vi "Replace Analysis Cluster.vi"() -> (0 "error out":errorcluster, 4 "Path":path)   [LabVIEW 2020]
panel:
  in  "OK Button":bool
  in  "stop":bool
  out "String":string
  in  "Correct Meas setup file":path
  in  "Analysis Cluster to Inject":string[][](array[string])=[["Inst Array", "Port", "Inst type", "Units symbol", "Sampling Rate (Hz)", "Device ID", "Sync Delay (ms)", "Ch No", "Use latest Calib", "Calib filename", "Label", "X Pos", "Y Pos", "Z Pos", "Initial X", "Initial Y", "Initial Z", "Traverse Setup", "On Axes", "ADAM_Ch_Name", "Code name", "Metadata Ch Names", "Metadata Ch Values"], ["LDA", "", "LDA Vel", "U", "250.00", "LDA_IP.vi", "0.00", "0", "FALSE", "", "", "80.000", "0.000", "-105.002", "0.000", "0.000", "0.000", "Aero_Enclosure", "X Y Z", "", "1LDA:U", "", ""], ["LDA", "", "LDA Vel", "W", "250.00", "LDA_IP.vi", "0.00", "1", "FALSE", "", "", "0.000", "0.000", "0.000", "0.000", "0.000", "0.000", "Position N/A", "X Y Z", "", "2LDA:U", "", ""], ["Analogue", "COM18", "Raw with zero offsetting", "N01", "800.00", "Pressure_Multiplexer.vi", "0.00", "0", "FALSE", "", "N01", "0.000", "0.000", "1.000", "0.000", "0.000", "1.000", "No Traverse", "X Y Z", "", "1RZ:U", "", ""], ["Analogue", "COM18", "Raw with zero offsetting", "N02", "800.00", "Pressure_Multiplexer.vi", "0.00", "1", "FALSE", "", "N02", "0.004", "0.013", "1.000", "0.004", "0.013", "1.000", "No Traverse", "X Y Z", "", "2RZ:U", "", ""], ["Analogue", "COM18", "Raw with zero offsetting", "N04", "800.00", "Pressure_Multiplexer.vi", "0.00", "2", "FALSE", "", "N04", "0.015", "0.025", "1.000", "0.015", "0.025", "1.000", "No Traverse", "X Y Z", "", "3RZ:U", "", ""], ["Analogue", "COM18", "Raw with zero offsetting", "N06", "800.00", "Pressure_Multiplexer.vi", "0.00", "3", "FALSE", "", "N06", "0.032", "0.037", "1.000", "0.032", "0.037", "1.000", "No Traverse", "X Y Z", "", "4RZ:U", "", ""], ["Analogue", "COM18", "Raw with zero offsetting", "N07", "800.00", "Pressure_Multiplexer.vi", "0.00", "4", "FALSE", "", "N07", "0.057", "0.047", "1.000", "0.057", "0.047", "1.000", "No Traverse", "X Y Z", "", "5RZ:U", "", ""], ["Analogue", "COM18", "Raw with zero offsetting", "N09", "800.00", "Pressure_Multiplexer.vi", "0.00", "5", "FALSE", "", "N09", "0.089", "0.056", "1.000", "0.089", "0.056", "1.000", "No Traverse", "X Y Z", "", "6RZ:U", "", ""], ["Analogue", "COM18", "Raw with zero offsetting", "N10", "800.00", "Pressure_Multiplexer.vi", "0.00", "6", "FALSE", "", "N10", "0.126", "0.063", "1.000", "0.126", "0.063", "1.000", "No Traverse", "X Y Z", "", "7RZ:U", "", ""], ["Analogue", "COM18", "Raw with zero offsetting", "N11", "800.00", "Pressure_Multiplexer.vi", "0.00", "7", "FALSE", "", "N11", "0.168", "0.069", "1.000", "0.168", "0.069", "1.000", "No Traverse", "X Y Z", "", "8RZ:U", "", ""], ["Analogue", "COM18", "Raw with zero offsetting", "N13", "800.00", "Pressure_Multiplexer.vi", "0.00", "8", "FALSE", "", "N13", "0.216", "0.073", "1.000", "0.216", "0.073", "1.000", "No Traverse", "X Y Z", "", "9RZ:U", "", ""], ["Analogue", "COM18", "Raw with zero offsetting", "N14", "800.00", "Pressure_Multiplexer.vi", "0.00", "34", "FALSE", "", "N14", "0.268", "0.075", "1.000", "0.268", "0.075", "1.000", "No Traverse", "X Y Z", "", "10RZ:U", "", ""], ["Analogue", "COM18", "Raw with zero offsetting", "N15", "800.00", "Pressure_Multiplexer.vi", "0.00", "10", "FALSE", "", "N15", "0.323", "0.075", "1.000", "0.323", "0.075", "1.000", "No Traverse", "X Y Z", "", "11RZ:U", "", ""], ["Analogue", "COM18", "Raw with zero offsetting", "N16", "800.00", "Pressure_Multiplexer.vi", "0.00", "11", "FALSE", "", "N16", "0.380", "0.073", "1.000", "0.380", "0.073", "1.000", "No Traverse", "X Y Z", "", "12RZ:U", "", ""], ["Analogue", "COM18", "Raw with zero offsetting", "N18", "800.00", "Pressure_Multiplexer.vi", "0.00", "12", "FALSE", "", "N18", "0.440", "0.070", "1.000", "0.440", "0.070", "1.000", "No Traverse", "X Y Z", "", "13RZ:U", "", ""], ["Analogue", "COM18", "Raw with zero offsetting", "N19", "800.00", "Pressure_Multiplexer.vi", "0.00", "13", "FALSE", "", "N19", "0.500", "0.066", "1.000", "0.500", "0.066", "1.000", "No Traverse", "X Y Z", "", "14RZ:U", "", ""], ["Analogue", "COM18", "Raw with zero offsetting", "N20", "800.00", "Pressure_Multiplexer.vi", "0.00", "14", "FALSE", "", "N20", "0.587", "0.058", "1.000", "0.587", "0.058", "1.000", "No Traverse", "X Y Z", "", "15RZ:U", "", ""], ["Analogue", "COM18", "Raw with zero offsetting", "N22", "800.00", "Pressure_Multiplexer.vi", "0.00", "15", "FALSE", "", "N22", "0.671", "0.049", "1.000", "0.671", "0.049", "1.000", "No Traverse", "X Y Z", "", "16RZ:U", "", ""], ["Analogue", "COM18", "Raw with zero offsetting", "N23", "800.00", "Pressure_Multiplexer.vi", "0.00", "16", "FALSE", "", "N23", "0.750", "0.040", "1.000", "0.750", "0.040", "1.000", "No Traverse", "X Y Z", "", "17RZ:U", "", ""], ["Analogue", "COM18", "Raw with zero offsetting", "N24", "800.00", "Pressure_Multiplexer.vi", "0.00", "17", "FALSE", "", "N24", "0.821", "0.030", "1.000", "0.821", "0.030", "1.000", "No Traverse", "X Y Z", "", "18RZ:U", "", ""], ["Analogue", "COM18", "Raw with zero offsetting", "N26", "800.00", "Pressure_Multiplexer.vi", "0.00", "18", "FALSE", "", "N26", "0.883", "0.021", "1.000", "0.883", "0.021", "1.000", "No Traverse", "X Y Z", "", "19RZ:U", "", ""], ["Analogue", "COM18", "Raw with zero offsetting", "N27", "800.00", "Pressure_Multiplexer.vi", "0.00", "19", "FALSE", "", "N27", "0.933", "0.013", "1.000", "0.933", "0.013", "1.000", "No Traverse", "X Y Z", "", "20RZ:U", "", ""], ["Analogue", "COM18", "Raw with zero offsetting", "N29", "800.00", "Pressure_Multiplexer.vi", "0.00", "20", "FALSE", "", "N29", "0.970", "0.007", "1.000", "0.970", "0.007", "1.000", "No Traverse", "X Y Z", "", "21RZ:U", "", ""], ["Analogue", "COM18", "Raw with zero offsetting", "N30", "800.00", "Pressure_Multiplexer.vi", "0.00", "21", "FALSE", "", "N30", "1.000", "0.000", "1.000", "1.000", "0.000", "1.000", "No Traverse", "X Y Z", "", "22RZ:U", "", ""], ["Analogue", "COM18", "Raw with zero offsetting", "N28", "800.00", "Pressure_Multiplexer.vi", "0.00", "22", "FALSE", "", "N28", "0.953", "-0.010", "-1.000", "0.953", "-0.010", "-1.000", "No Traverse", "X Y Z", "", "23RZ:U", "", ""], ["Analogue", "COM18", "Raw with zero offsetting", "N25", "800.00", "Pressure_Multiplexer.vi", "0.00", "23", "FALSE", "", "N25", "0.821", "-0.030", "-1.000", "0.821", "-0.030", "-1.000", "No Traverse", "X Y Z", "", "24RZ:U", "", ""], ["Analogue", "COM18", "Raw with zero offsetting", "N21", "800.00", "Pressure_Multiplexer.vi", "0.00", "24", "FALSE", "", "N21", "0.629", "-0.054", "-1.000", "0.629", "-0.054", "-1.000", "No Traverse", "X Y Z", "", "25RZ:U", "", ""], ["Analogue", "COM18", "Raw with zero offsetting", "N17", "800.00", "Pressure_Multiplexer.vi", "0.00", "25", "FALSE", "", "N17", "0.413", "-0.072", "-1.000", "0.413", "-0.072", "-1.000", "No Traverse", "X Y Z", "", "26RZ:U", "", ""], ["Analogue", "COM18", "Raw with zero offsetting", "N12", "800.00", "Pressure_Multiplexer.vi", "0.00", "26", "FALSE", "", "N12", "0.213", "-0.073", "-1.000", "0.213", "-0.073", "-1.000", "No Traverse", "X Y Z", "", "27RZ:U", "", ""], ["Analogue", "COM18", "Raw with zero offsetting", "N08", "800.00", "Pressure_Multiplexer.vi", "0.00", "27", "FALSE", "", "N08", "0.067", "-0.050", "-1.000", "0.067", "-0.050", "-1.000", "No Traverse", "X Y Z", "", "28RZ:U", "", ""], ["Analogue", "COM18", "Raw with zero offsetting", "N05", "800.00", "Pressure_Multiplexer.vi", "0.00", "28", "FALSE", "", "N05", "0.021", "-0.030", "-1.000", "0.021", "-0.030", "-1.000", "No Traverse", "X Y Z", "", "29RZ:U", "", ""], ["Analogue", "COM18", "Raw with zero offsetting", "N03", "800.00", "Pressure_Multiplexer.vi", "0.00", "29", "FALSE", "", "N03", "0.004", "-0.014", "-1.000", "0.004", "-0.014", "-1.000", "No Traverse", "X Y Z", "", "30RZ:U", "", ""], ["Analogue", "COM23", "Generic Polynomial", "D", "5000.00", "Na-DAS_7609.vi", "0.00", "0", "FALSE", "Z:\\2021\\Aero_Tunnel\\Haydn Wootton\\Calibrations\\Cal_12-2021\\Laser Disp Volts to Angle2.xls", "", "0.000", "0.000", "0.000", "0.000", "0.000", "0.000", "Position N/A", "X Y Z", "", "1Gen:U", "", ""], ["Analogue", "COM23", "Raw voltage", "Sync", "5000.00", "Na-DAS_7609.vi", "0.00", "1", "FALSE", "", "", "0.000", "0.000", "0.000", "0.000", "0.000", "0.000", "Position N/A", "X Y Z", "", "1RV:U", "", ""]]
  out "Array":path[](array[path])
  out "File Changed":bool
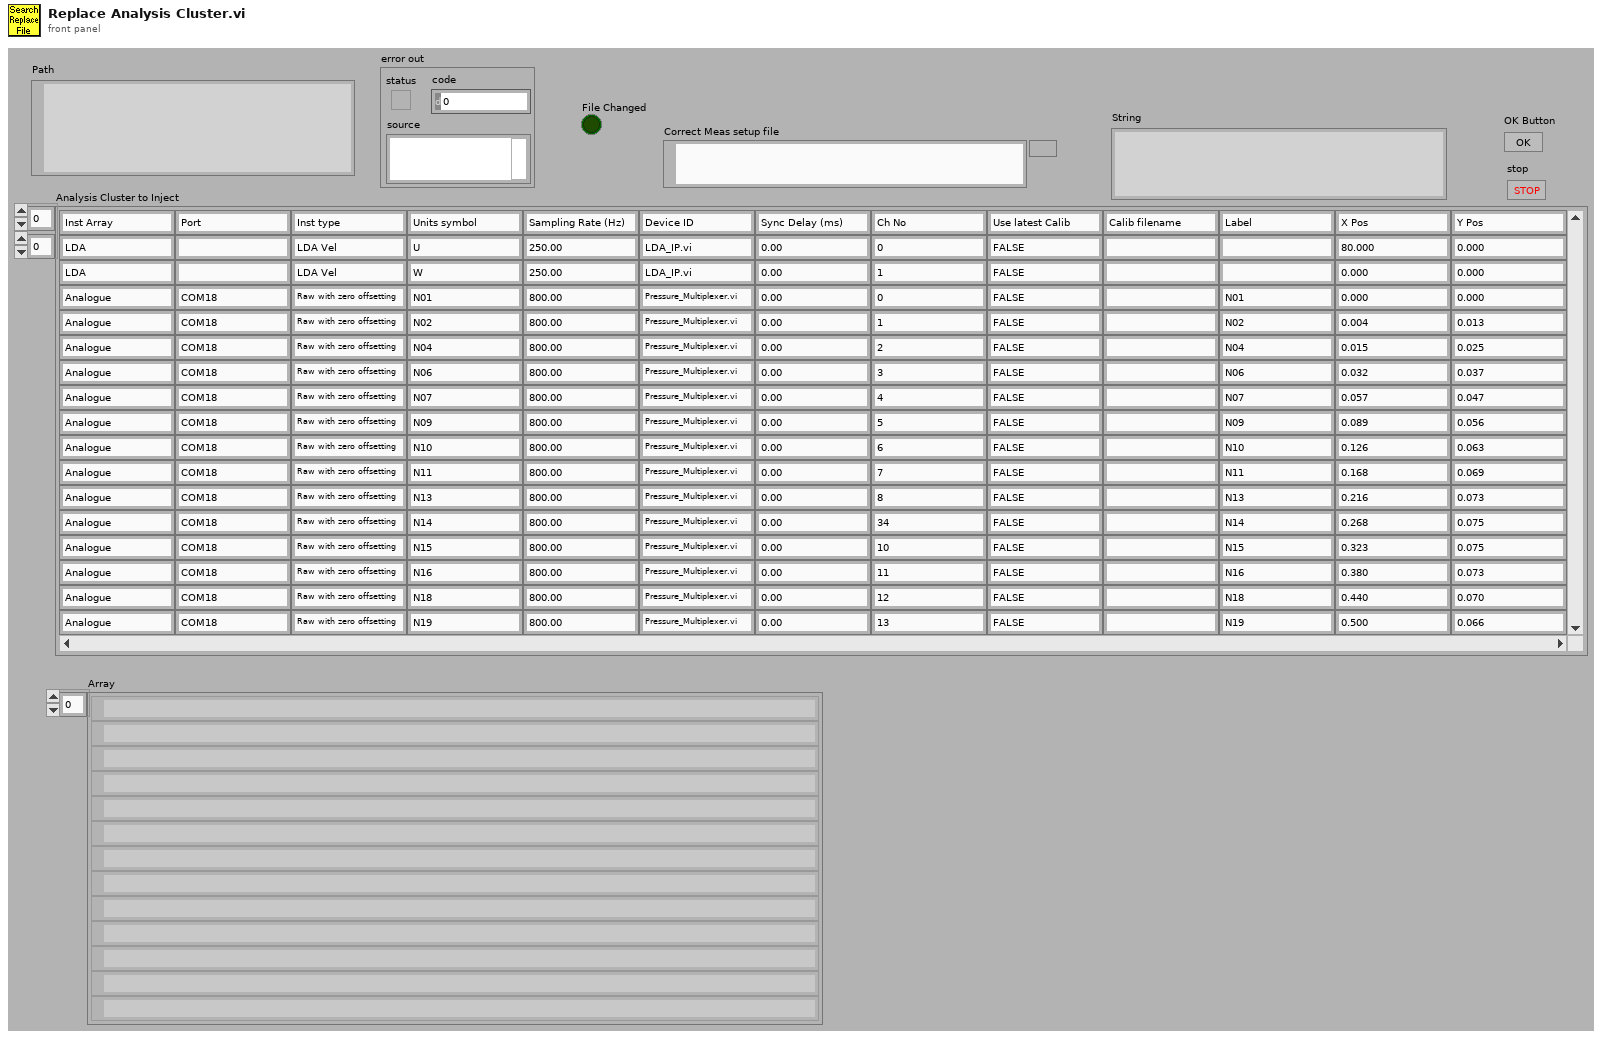
[diagram p1: front panel]
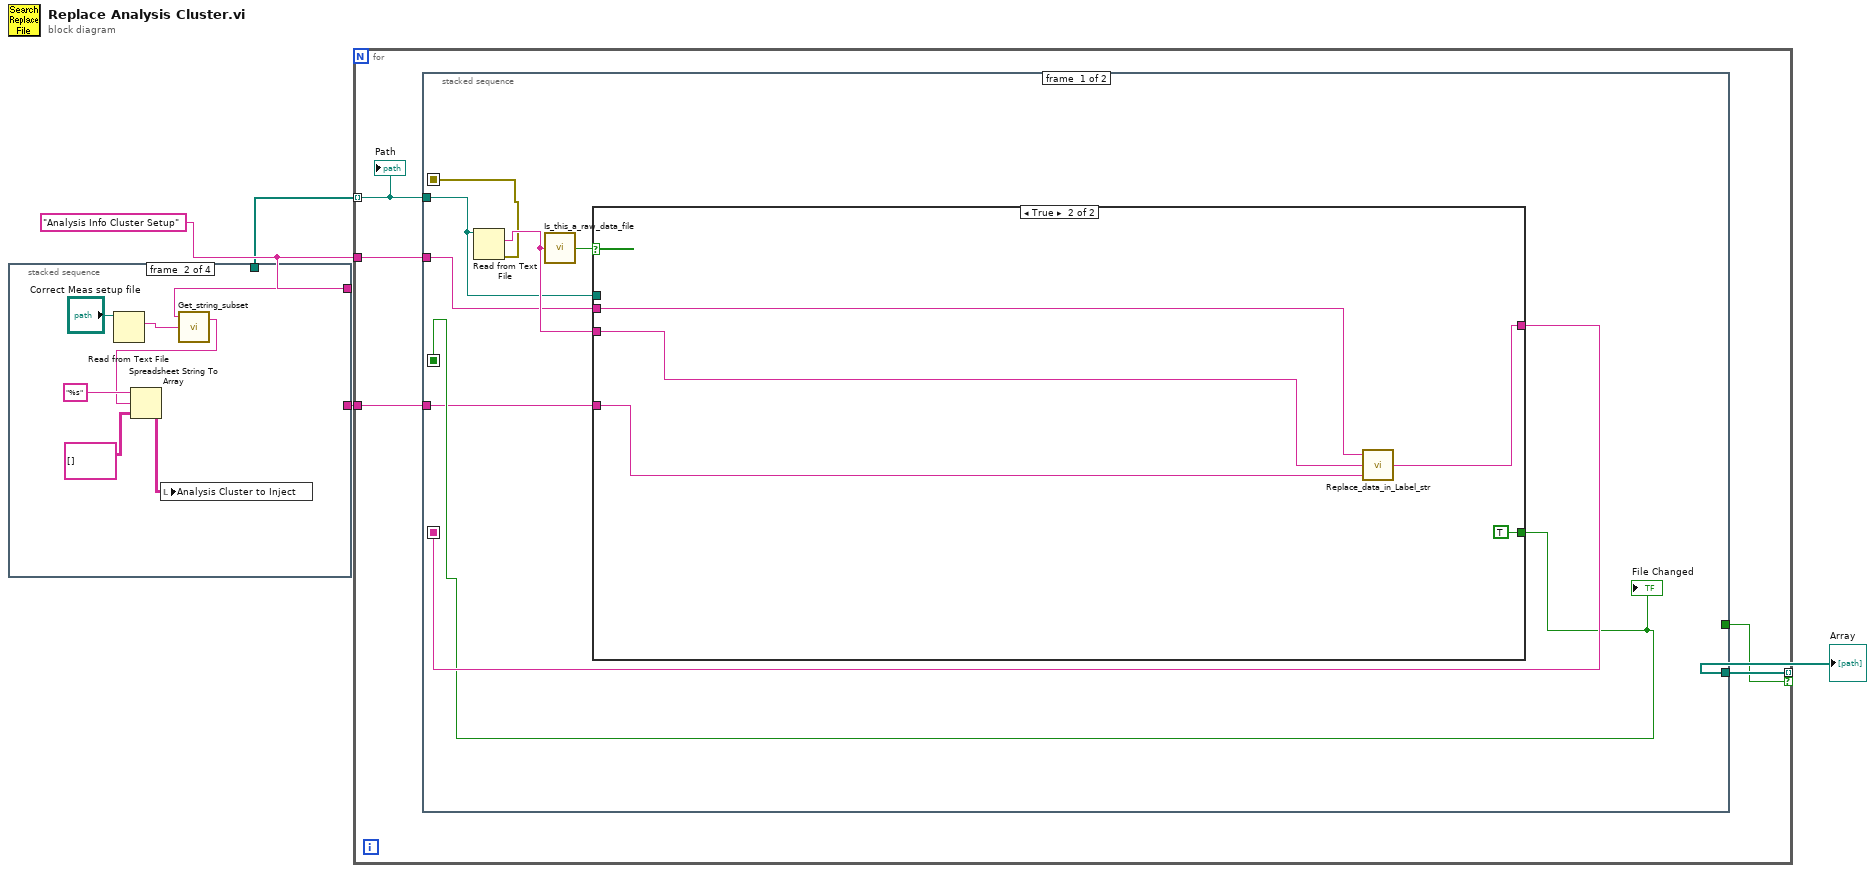
[diagram p0: block diagram]
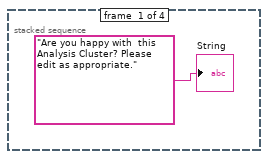
[diagram p2: hidden frame]
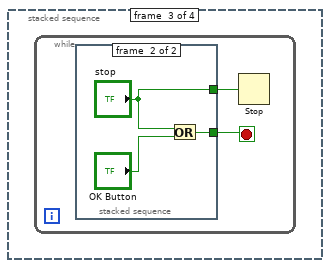
[diagram p3: hidden frame]
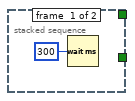
[diagram p4: hidden frame]
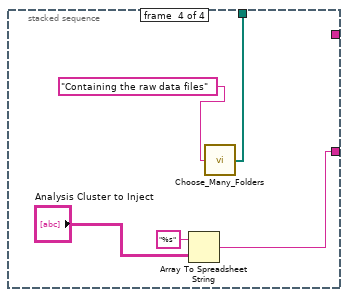
[diagram p5: hidden frame]
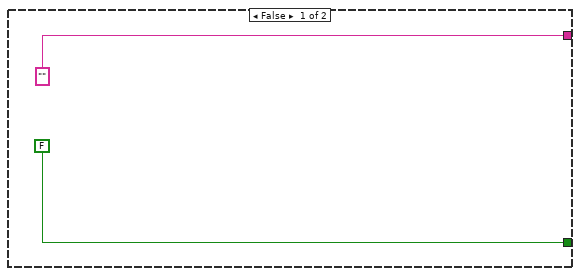
[diagram p6: hidden frame]
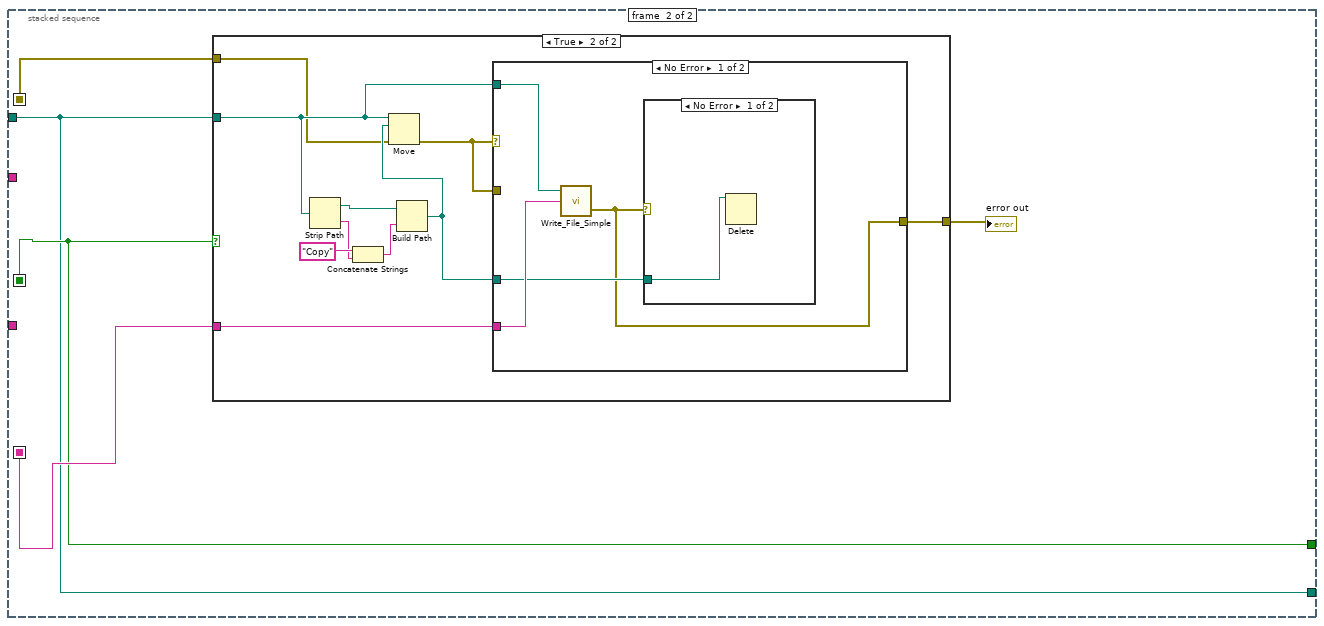
[diagram p7: hidden frame]
diagram:
  w3 = "Analysis Info Cluster Setup"
  n1 = stacked-sequence {
    tunnel: w3 -> [_ w11 _ _]
    tunnel: [_ _ _ w19] -> w2
    tunnel: [_ _ _ w22] -> w1
    frame #0 {
      "String" <- "Are you happy with  this Analysis Cluster? Please edit as appropriate."
    }
    frame #1 {
      n2 = Read from Text File(file (use dialog)="Correct Meas setup file") -> (text=w12:string)  [unwired: 3 in, 3 out]
      n3 = call "Get_string_subset.vi"("String to split"=w12, "File Label"=w11) -> ("Output string"=w7:string)  [unwired: 2 in, 1 out]
      n4 = Spreadsheet String To Array(format string="%s", spreadsheet string=w7, array type (2D Dbl)=string[][] []) -> (array=w6:string[][])  [unwired: 1 in]
      n5 = local write "Analysis Cluster to Inject"(w6) -> ()
    }
    frame #2 {
      n6 = while {
        stop <- w14 stop-if-true
        n7 = stacked-sequence {
          tunnel: [_ w17] -> w14
          tunnel: [_ "stop"] -> w13
          frame #0 {
            n8 = Wait (ms)(milliseconds to wait=u32 300) -> ()  [unwired: 1 out]
          }
          frame #1 {
            n9 = Or(x="stop", y="OK Button") -> (x .or. y?=w17:bool)
          }
        }
        n10 = Stop(stop? (T)=w13) -> ()
      }
    }
    frame #3 {
      n11 = Array To Spreadsheet String(array="Analysis Cluster to Inject", 3:"%s" ("format string")) -> (spreadsheet string=w19:string)  [unwired: 1 in]
      n12 = call "Choose_Many_Folders.vi"("Purpose of choosing folder"="Containing the raw data files") -> ("Files"=w22:path[])
    }
  }
  n13 = for {
    tunnel: w1 -> [w28] mode=indexing
    tunnel: [w27] -> w4 mode=indexing if=w26
    tunnel: w3 -> [w25]
    tunnel: w2 -> [w24]
    n14 = stacked-sequence {
      seq-local: [w32 _] -> [_ w47]
      seq-local: [w36 _] -> [_ w46]
      seq-local: [w35 _] -> [_ w45]
      tunnel: w28 -> [w31 w44]
      tunnel: [_ w44] -> w27
      tunnel: [_ w45] -> w26
      tunnel: w25 -> [w30 _]
      tunnel: w24 -> [w29 _]
      frame #0 {
        n15 = Read from Text File(file (use dialog)=w31) -> (text=w33:string, error out=w32:errorcluster)  [unwired: 3 in, 2 out]
        n16 = call "Is_this_a_raw_data_file.vi"("character string"=w33) -> ("Raw Dat File?"=w34:bool)  [unwired: 2 out]
        n17 = case shown="True" w34 {
          tunnel: ["" ("string") w42] -> w36
          tunnel: [FALSE TRUE] -> w35
          tunnel: w33 -> [_ w43]
          tunnel: w31 -> [_ _]
          tunnel: w30 -> [_ w41]
          tunnel: w29 -> [_ w40]
          frame False {
          }
          frame True {
            n18 = call "Replace_data_in_Label_str.vi"("New data string"=w40, "Input string"=w43, "Variable name"=w41) -> ("Appended string"=w42:string)
          }
        }
        "File Changed" <- w35
      }
      frame #1 {
        n19 = case shown="True" w45 {
          tunnel: w44 -> [_ w55]
          tunnel: w46 -> [_ w54]
          tunnel: [w49 w52] -> w48
          tunnel: w47 -> [w49 w50]
          frame False {
          }
          frame True {
            n20 = Strip Path(path=w55) -> (stripped path=w56:path, name=w58:string)
            n21 = Concatenate Strings("Copy" ("name or relative path"), w58) -> (w57:string)
            n22 = Build Path(base path=w56, name or relative path=w57) -> (appended path=w53:path)
            n23 = Move(source path=w55, error in=w50, 10:w53) -> (error out=w51:errorcluster)  [unwired: 2 in, 2 out]
            n24 = case shown="No Error" w51 {
              tunnel: w55 -> [w63 _]
              tunnel: w54 -> [w62 _]
              tunnel: w53 -> [w61 _]
              tunnel: [w60 w65] -> w52
              tunnel: w51 -> [_ w65]
              frame No Error {
                n25 = call "Write_File_Simple.vi"("character string"=w62, "file path"=w63) -> ("error out"=w60:errorcluster)  [unwired: 1 in, 1 out]
                n26 = case shown="No Error" w60 {
                  tunnel: w61 -> [w64 _]
                  frame No Error {
                    n27 = Delete(path (use dialog)=w64) -> ()  [unwired: 4 in, 3 out]
                  }
                  frame Error {
                  }
                }
              }
              frame Error {
              }
            }
          }
        }
        "error out" <- w48
      }
    }
    "Path" <- w28
  }
  "Array" <- w4
